vi "sorter.vi"() -> ()   [LabVIEW 2016]
uses:
  <vilib>/vision/NI_Vision_Development_Module.lvlib
panel:
  in  "reset":bool
  out "Slide":dbl(slide) scale=0.0..50.0
  out "motor":bool
  out "green":bool
  out "red":bool
  out "sensor":bool
  out "stop":bool
  out "start":bool
  out "Color Spectrum":dbl[](array[numeric]) format="%.2f"
  in  "Stop (F)":bool
  out "Image Out":T1(plugin-control)
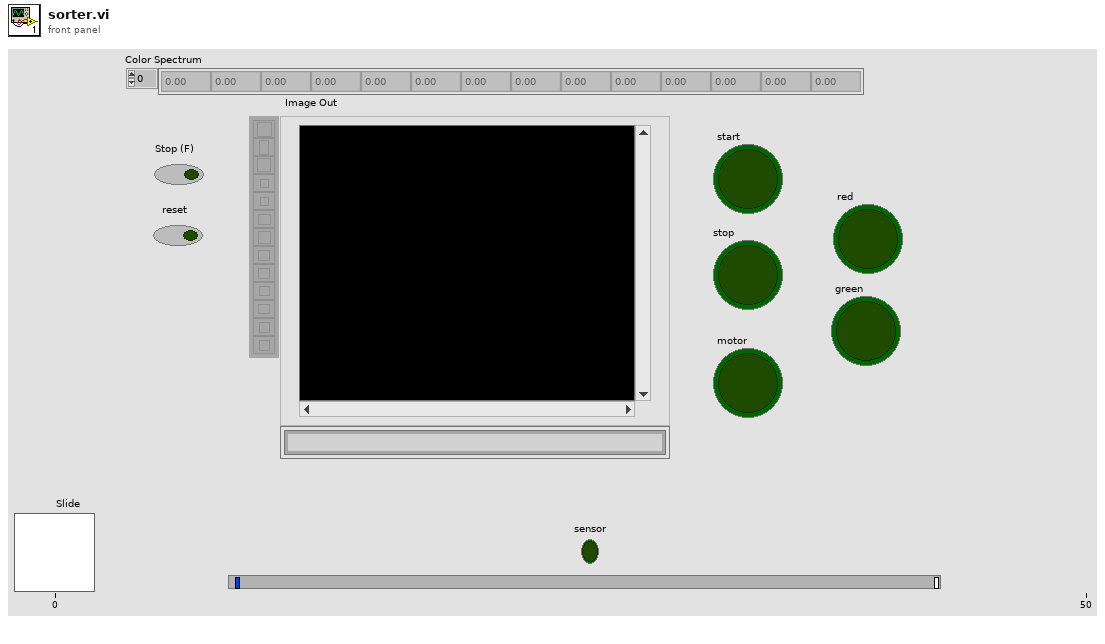
[diagram p1: front panel]
types:
  T1 = typedef "IMAQ Image.ctl" = refnum<image>
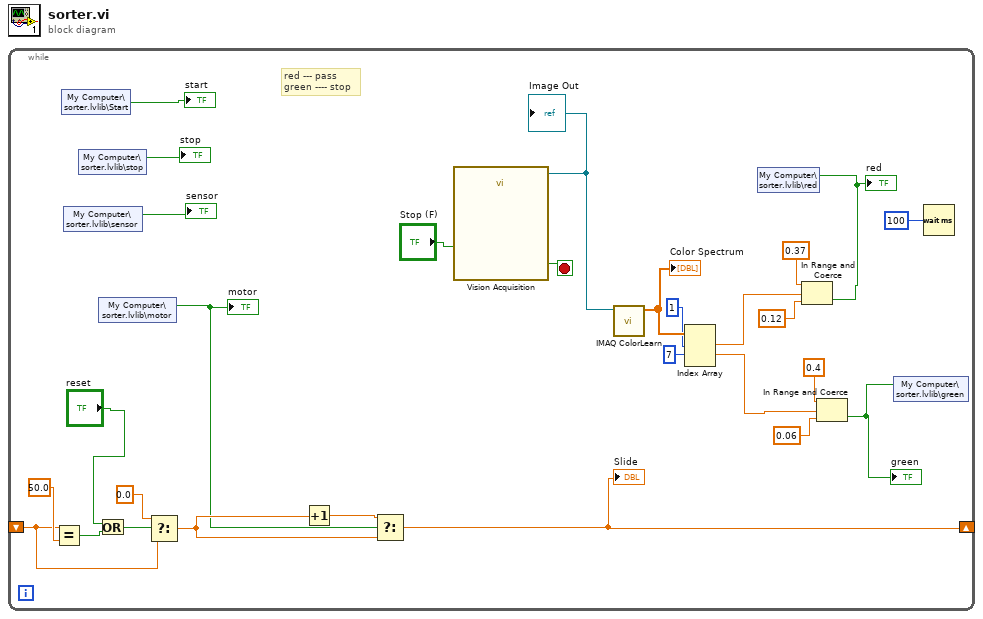
[diagram p0: block diagram]
diagram:
  n1 = while {
    shift-right: [w14] -> _
    shift-left: _ -> [w11]
    stop <- w16 stop-if-true
    # "red --- pass \ngreen ---- stop"
    n2 = Equal?(x=w11, y=50.0) -> (x = y?=w8:bool)
    n3 = shared-variable "My Computer\\sorter.lvlib\\Start"() -> (→"start":bool)  [unwired: 1 in, 1 out]
    n4 = shared-variable "My Computer\\sorter.lvlib\\sensor"() -> (→"sensor":bool)  [unwired: 1 in, 1 out]
    n5 = shared-variable "My Computer\\sorter.lvlib\\stop"() -> (→"stop":bool)  [unwired: 1 in, 1 out]
    n6 = Or(x="reset", y=w8) -> (x .or. y?=w9:bool)
    n7 = shared-variable "My Computer\\sorter.lvlib\\motor"() -> (w6:bool)  [unwired: 1 in, 1 out]
    "motor" <- w6
    n8 = Select(t=0.0, s=w9, f=w11) -> (s? t:f=w10:dbl)
    n9 = Increment(x=w10) -> (x+1=w15:dbl)
    n10 = Select(t=w15, s=w6, f=w10) -> (s? t:f=w14:dbl)
    "Slide" <- w14
    n11 = call "Vision Acquisition"("Stop (F)"="Stop (F)") -> ("Image Out"=w27:T1, "Stopped"=w16:bool)  [unwired: 24 in, 1 out]
    "Image Out" <- w27
    n12 = call "IMAQ ColorLearn"("Image"=w27) -> ("Color Spectrum"=w26:dbl[])  [unwired: 7 in, 1 out]
    "Color Spectrum" <- w26
    n13 = Index Array(array=w26, index #1=1 ("index"), index #2=7 ("index")) -> (element #1=w24:dbl, element #2=w18:dbl)  [unwired: 1 in, 1 out]
    n14 = In Range and Coerce(upper limit=0.37, x=w24, lower limit=0.12) -> (In Range?=w4:bool)  [unwired: 1 out]
    "red" <- w4
    n15 = shared-variable "My Computer\\sorter.lvlib\\red"(w4) -> ()  [unwired: 1 in, 1 out]
    n16 = In Range and Coerce(upper limit=0.4, x=w18, lower limit=0.06) -> (In Range?=w3:bool)  [unwired: 1 out]
    "green" <- w3
    n17 = shared-variable "My Computer\\sorter.lvlib\\green"(w3) -> ()  [unwired: 1 in, 1 out]
    n18 = Wait (ms)(milliseconds to wait=u32 100 ("millisecond multiple")) -> ()  [unwired: 1 out]
  }
